vi "SequenceIndexWriteUI.vi"(10 "SequenceIndexFill":refnum<class "SequenceIndex.lvclass">, 11 "VariableManagerRef in":refnum<vi>) -> (2 "SequenceIndexWrote":refnum<class "SequenceIndex.lvclass">, 3 "VariableManagerRef out":refnum<vi>)   [LabVIEW 2013]
doc: "Create a window for add/edit sequence index of the given VariableManager reference. SequenceIndexWrote is returned when the user successfully add/edit the sequence index. SequenceIndexWrote has empty name if the user cancel the operation.\n\nThe name of SequenceIndexFill will determine the operation. \nIf the name of SequenceIndexFill already exists, the operation is editing the sequence index.\nIf the name of SequenceIndexFill does not exists, the operation is adding a new sequence index."
uses:
  VariableManager/VariableManager.lvclass
  SequenceIndex/SequenceIndex.lvclass
  API/VariableManagerAPI.lvlib
panel:
  in  "Steps":u32=1
  in  "SequenceIndexName":string
  out "Operation":string
  in  "OK Button":bool
  in  "Cancel Button":bool
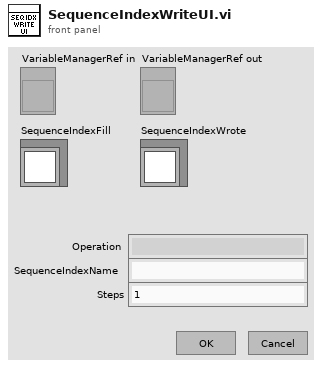
[diagram p1: front panel]
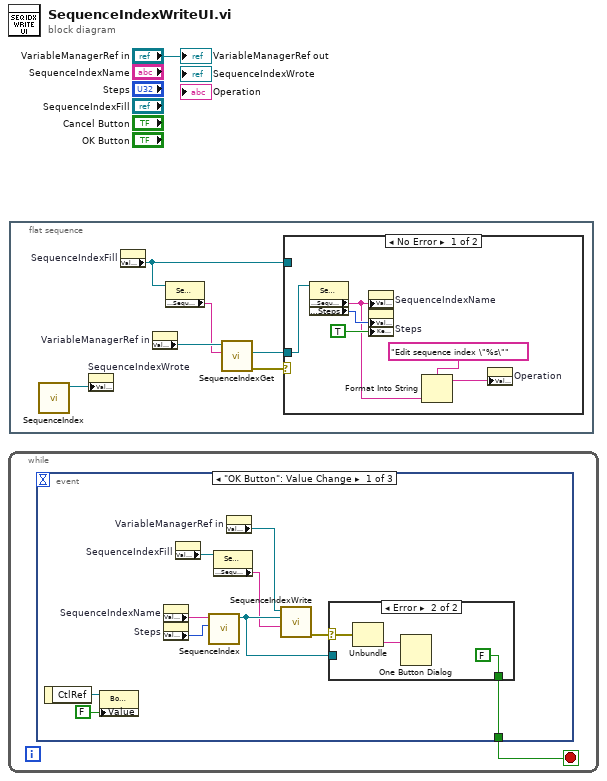
[diagram p0: block diagram]
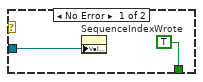
[diagram p2: hidden frame]
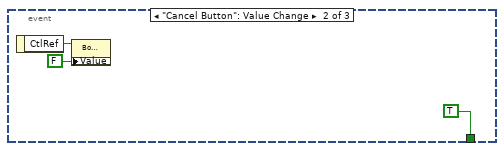
[diagram p3: hidden frame]
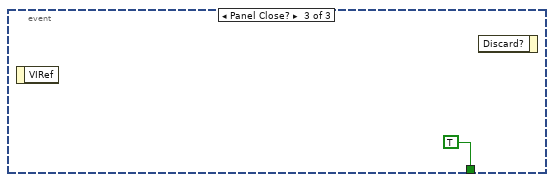
[diagram p4: hidden frame]
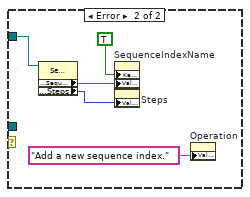
[diagram p5: hidden frame]
diagram:
  n1 = while {
    stop <- w2 stop-if-true
    n2 = event shown="[0] \"OK Button\": Value Change" {
      selector: _ -> [_ _ _]
      dyn-events: _ -> [_ _ _]
      timeout: _ -> [_ _ _]
      tunnel: [w10 TRUE TRUE] -> w2
      event "OK Button": Value Change {
        n3 = event-data() -> ("CtlRef"=w12:refnum<vi>)  [unwired: 1 in]
        n4 = property class="Bool (strict)"(reference=w12, "Value"=FALSE) -> ()  [unwired: 1 in, 2 out]
        n5 = property on="SequenceIndexName" class="Str"() -> ("Value"=w4:string)  [unwired: 2 in, 2 out]
        n6 = property on="Steps" class="DigNum (strict)"() -> ("Value"=w3:u32)  [unwired: 2 in, 2 out]
        n7 = property on="SequenceIndexFill" class="LVClassControl (strict)"() -> ("Value"=w9:refnum<class "SequenceIndex.lvclass">)  [unwired: 2 in, 2 out]
        n8 = call "SequenceIndex.vi"("Steps"=w3, "SequenceIndexName"=w4) -> ("SequenceIndex"=w7:refnum<class "SequenceIndex.lvclass">)  [unwired: 9 in]
        n9 = property class="SequenceIndex.lvclass"(reference=w9) -> ("Accessors:SequenceIndexName"=w6:string)  [unwired: 1 in, 2 out]
        n10 = property on="VariableManagerRef in" class="LVObjRef (strict)"() -> ("Value"=w8:refnum<vi>)  [unwired: 2 in, 2 out]
        n11 = call "SequenceIndexWrite.vi"("OriginalName"=w6, "SequenceIndex"=w7, "VariableManagerRef in"=w8) -> ("error out"=w5:errorcluster)  [unwired: 7 in, 1 out]
        n12 = case shown="Error" w5 {
          selector: w5 -> [_ w16]
          tunnel: [TRUE FALSE] -> w10
          tunnel: w7 -> [w13 _]
          frame No Error {
            n13 = property on="SequenceIndexWrote" class="LVClassControl (strict)"("Value"=w13) -> ()  [unwired: 2 in, 2 out]
          }
          frame Error {
            n14 = Unbundle(w16) -> ("source"=w15:string)  [unwired: 2 out]
            n15 = One Button Dialog(message=w15) -> ()  [unwired: 1 in, 1 out]
          }
        }
      }
      event "Cancel Button": Value Change {
        n16 = event-data() -> ("CtlRef"=w19:refnum<vi>)  [unwired: 1 in]
        n17 = property class="Bool (strict)"(reference=w19, "Value"=FALSE) -> ()  [unwired: 1 in, 2 out]
      }
      event Panel Close? {
        n18 = event-data() -> ()  [unwired: 1 in, 1 out]
        n19 = event-data() -> ()  [unwired: 2 in, 1 out]
      }
    }
  }
  n20 = flat-sequence {
    frame #0 {
      n21 = call "SequenceIndex.vi"() -> ("SequenceIndex"=w22:refnum<class "SequenceIndex.lvclass">)  [unwired: 11 in]
      n22 = property on="SequenceIndexWrote" class="LVClassControl (strict)"("Value"=w22) -> ()  [unwired: 2 in, 2 out]
      n23 = property on="SequenceIndexFill" class="LVClassControl (strict)"() -> ("Value"=w23:refnum<class "SequenceIndex.lvclass">)  [unwired: 2 in, 2 out]
      n24 = property on="VariableManagerRef in" class="LVObjRef (strict)"() -> ("Value"=w27:refnum<vi>)  [unwired: 2 in, 2 out]
      n25 = property class="SequenceIndex.lvclass"(reference=w23) -> ("Accessors:SequenceIndexName"=w26:string)  [unwired: 1 in, 2 out]
      n26 = call "SequenceIndexGet.vi"("SequenceIndexName"=w26, "VariableManagerRef in"=w27) -> ("error out"=w24:errorcluster, "SequenceIndex"=w25:refnum<class "SequenceIndex.lvclass">)  [unwired: 7 in, 1 out]
      n27 = case shown="No Error" w24 {
        tunnel: w25 -> [w33 _]
        tunnel: w23 -> [_ w38]
        frame No Error {
          n28 = property class="SequenceIndex.lvclass"(reference=w33) -> ("Accessors:SequenceIndexName"=w28:string, "Accessors:Steps"=w29:u32)  [unwired: 1 in, 2 out]
          n29 = property on="SequenceIndexName" class="Str"("Value"=w28) -> ()  [unwired: 2 in, 2 out]
          n30 = property on="Steps" class="DigNum (strict)"("Value"=w29, "Key Focus"=TRUE) -> ()  [unwired: 2 in, 2 out]
          n31 = Format Into String(format string="Edit sequence index \"%s\"", w28) -> (resulting string=w31:string)  [unwired: 2 in, 1 out]
          n32 = property on="Operation" class="Str"("Value"=w31) -> ()  [unwired: 2 in, 2 out]
        }
        frame Error {
          n33 = property class="SequenceIndex.lvclass"(reference=w38) -> ("Accessors:SequenceIndexName"=w36:string, "Accessors:Steps"=w35:u32)  [unwired: 1 in, 2 out]
          n34 = property on="SequenceIndexName" class="Str"("Key Focus"=TRUE, "Value"=w36) -> ()  [unwired: 2 in, 2 out]
          n35 = property on="Steps" class="DigNum (strict)"("Value"=w35) -> ()  [unwired: 2 in, 2 out]
          n36 = property on="Operation" class="Str"("Value"="Add a new sequence index.") -> ()  [unwired: 2 in, 2 out]
        }
      }
    }
  }
  "VariableManagerRef out" <- "VariableManagerRef in"
